vi "ZE_Recorder_FPelemVisible.vi"(8 "error in":errorcluster, 10 "Visible?":bool, 11 "FP Elems":refnum<vi>[](array[refnum])) -> (0 "error out":errorcluster, 3 "FP Elems out":refnum<vi>[](array[refnum]))   [LabVIEW 2025, in "ZE_Recorder.lvlib"]
doc: "ZE_Recorder_FPelemVisible.vi\n----------------------------------------------\nSets Front Page Elements to visible or invisible\n\nInputs:\n---------------------\nerror in: Cluster: \nVisible?: Boolean: \nFP Elems: Array: \n\n\nOutputs:\n---------------------\nerror out: Cluster: \nFP Elems out: Array: \n\n\n----------------------------------------------\n27.12.17\nZühlke Engineering AG\nCH-8952 Schlieren\nwww.zuehlke.com"
uses:
  ZE_Recorder.lvlib
panel:
  # "Connector Pane"
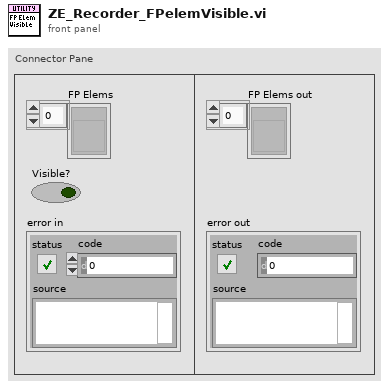
[diagram p1: front panel]
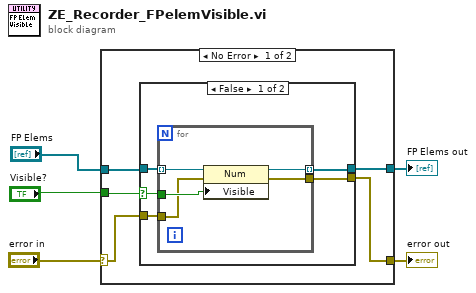
[diagram p0: block diagram]
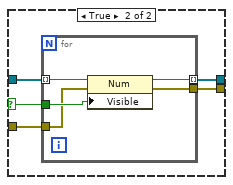
[diagram p2: hidden frame]
diagram:
  n1 = case shown="No Error" "error in" {
    selector: "error in" -> [w8 w32]
    tunnel: "Visible?" -> [w10 _]
    tunnel: "FP Elems" -> [w9 w31]
    tunnel: [w7 w32] -> w1
    tunnel: [w6 w31] -> w2
    frame No Error {
      n2 = case shown="False" w10 {
        selector: w10 -> [w14 w24]
        tunnel: w9 -> [w13 w25]
        tunnel: w8 -> [w15 w23]
        tunnel: [w11 w22] -> w7
        tunnel: [w12 w21] -> w6
        frame False {
          n3 = for {
            tunnel: w13 -> [w20] mode=indexing
            tunnel: w14 -> [w19]
            tunnel: w15 -> [w18]
            tunnel: [w17] -> w11
            tunnel: [w16] -> w12 mode=indexing
            n4 = property class="Num"(reference=w20, error in=w18, "Visible"=w19) -> (reference out=w16:refnum<vi>, error out=w17:errorcluster)
          }
        }
        frame True {
          n5 = for {
            tunnel: w25 -> [w30] mode=indexing
            tunnel: w24 -> [w29]
            tunnel: w23 -> [w28]
            tunnel: [w27] -> w22
            tunnel: [w26] -> w21 mode=indexing
            n6 = property class="Num"(reference=w30, error in=w28, "Visible"=w29) -> (reference out=w26:refnum<vi>, error out=w27:errorcluster)
          }
        }
      }
    }
    frame Error {
    }
  }
  "FP Elems out" <- w2
  "error out" <- w1
